vi "FindValidBuildSpecs.vi"(8 "error in (no error)":errorcluster, 9 "Target Name":string, 10 "ProjectItem Refnums":refnum<vi>[](array[refnum]), 11 "ExecuteAllBuildSpecs in":refnum<class "ExecuteAllBuildSpecs.lvclass">) -> (0 "error out":errorcluster, 1 "Specs":T1[](array[typedef]), 2 "dup ProjectItem Refnums":refnum<vi>[](array[refnum]), 3 "ExecuteAllBuildSpecs out":refnum<class "ExecuteAllBuildSpecs.lvclass">)   [LabVIEW 2014, in "ExecuteAllBuildSpecs.lvclass"]
doc: "Locates all build specs in the project."
uses:
  ExecuteAllBuildSpecs.lvclass
  ExecuteMultipleBuildSpecs/SpecInformation.ctl
  ExecuteMultipleBuildSpecs/ExecuteMultipleBuildSpecs.lvclass
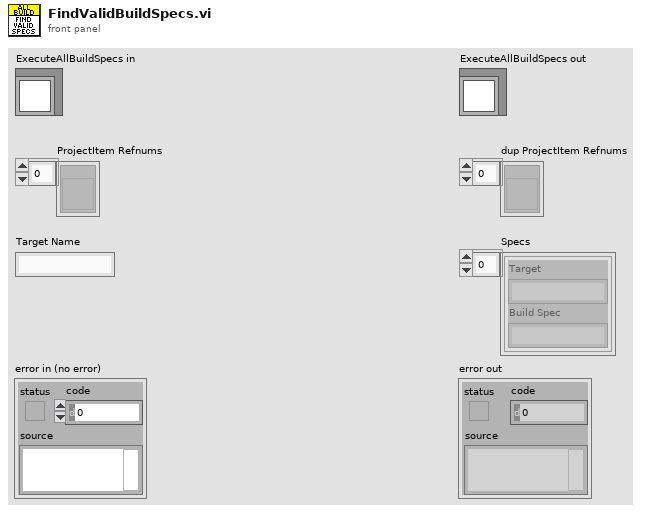
[diagram p1: front panel]
types:
  T1 = typedef "ExecuteMultipleBuildSpecs.lvclass/SpecInformation.ctl" = cluster{"Target":string, "Build Spec":string}
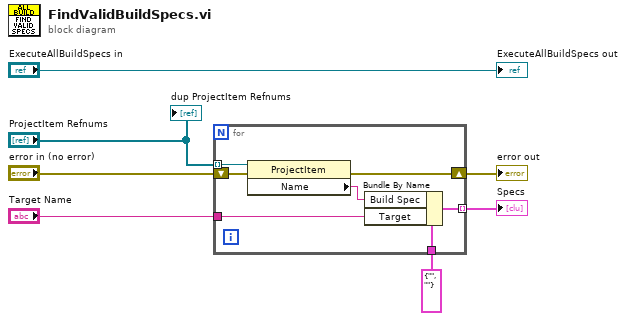
[diagram p0: block diagram]
diagram:
  n1 = for {
    tunnel: "ProjectItem Refnums" -> [w13] mode=indexing
    shift-right: [w12] -> w4
    shift-left: "error in (no error)" -> [w14]
    tunnel: "Target Name" -> [w9]
    tunnel: T1 {"Target"="", "Build Spec"=""} ("Spec Info") -> [w11]
    tunnel: [w8] -> w3 mode=indexing
    n2 = property class="ProjectItem"(reference=w13, error in=w14) -> (error out=w12:errorcluster, "Name"=w10:string)  [unwired: 1 out]
    n3 = Bundle By Name(cluster=w11, "Build Spec"=w10, "Target"=w9) -> (w8:T1)
  }
  "error out" <- w4
  "Specs" <- w3
  "ExecuteAllBuildSpecs out" <- "ExecuteAllBuildSpecs in"
  "dup ProjectItem Refnums" <- "ProjectItem Refnums"
